vi "SUB_ContinueCom1Read_new.vi"(3 "error out 2":errorcluster, 4 "Numeric":i32, 5 "duplicate VISA resource name 2":refnum<visa-resource-name>) -> (0 "error out":errorcluster, 1 "String":string, 2 "duplicate VISA resource name":refnum<visa-resource-name>)   [LabVIEW 2011]
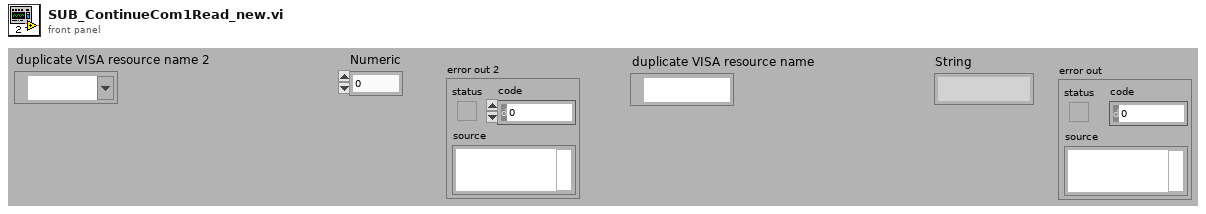
[diagram p1: front panel]
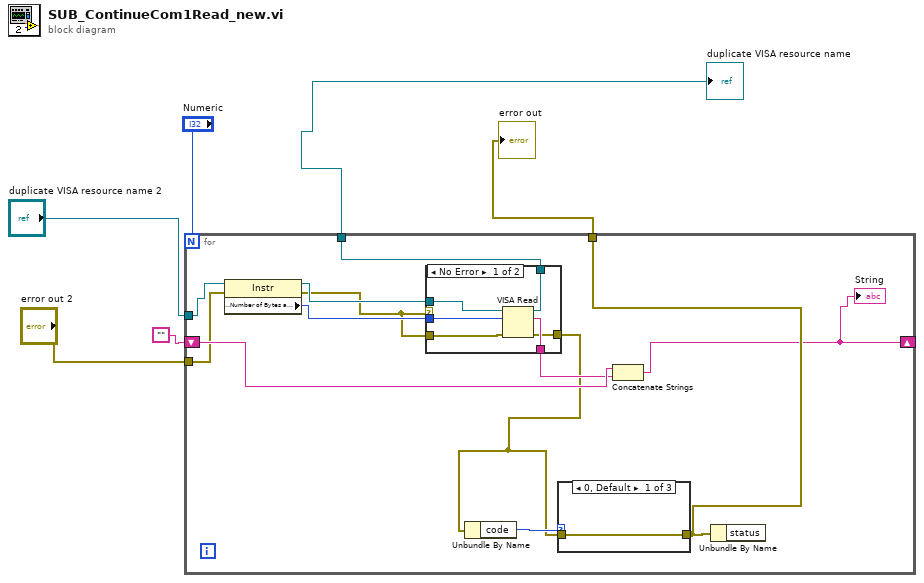
[diagram p0: block diagram]
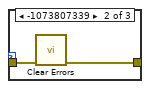
[diagram p2: hidden frame]
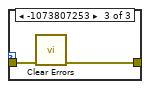
[diagram p3: hidden frame]
diagram:
  n1 = for {
    N: "Numeric" -> [_]
    shift-right: [w7] -> _
    shift-left: "" -> [w17]
    tunnel: "duplicate VISA resource name 2" -> [w14]
    tunnel: "error out 2" -> [w13]
    tunnel: [w15] -> w6
    tunnel: [w8] -> w1
    n2 = property class="Instr"(reference=w14, error in=w13) -> (reference out=w12:refnum<visa-resource-name>, error out=w11:errorcluster, "Serial Settings:Number of Bytes at Serial Port"=w18:u32)
    n3 = case shown="No Error" w11 {
      tunnel: w18 -> [w29 _]
      tunnel: [w28 _] -> w16
      tunnel: [w27 _] -> w15
      tunnel: w12 -> [w26 _]
      tunnel: [w25 w30] -> w9
      tunnel: w11 -> [w24 w30]
      frame No Error {
        n4 = VISA Read(VISA resource name=w26, byte count=w29, error in (no error)=w24) -> (VISA resource name out=w27:refnum<visa-resource-name>, read buffer=w28:string, error out=w25:errorcluster)  [unwired: 1 out]
      }
      frame Error {
      }
    }
    n5 = Unbundle By Name(w9) -> ("code"=w10:i32)
    n6 = case shown="0, Default" w10 {
      tunnel: w9 -> [w19 w21 w23]
      tunnel: [w19 w20 w22] -> w8
      frame 0, Default {
      }
      frame -1073807339 {
        n7 = call <vilib>:"Clear Errors.vi"("error in (no error)"=w21) -> ("error out"=w20:errorcluster)  [unwired: 6 in]
      }
      frame -1073807253 {
        n8 = call <vilib>:"Clear Errors.vi"("error in (no error)"=w23) -> ("error out"=w22:errorcluster)  [unwired: 6 in]
      }
    }
    n9 = Concatenate Strings(w17, w16) -> (w7:string)
    "String" <- w7
    n10 = Unbundle By Name(w8) -> ()  [unwired: 1 out]
  }
  "error out" <- w1
  "duplicate VISA resource name" <- w6
